vi "Measure vs B2Dv12.vi"() -> ()   [LabVIEW 2009]
doc: "This VI is an example operator panel.\n\nThe VI contains a table for the field values that may be configured manually, or loaded by checking the \"Prompt for File\" box. The data file should contain 3 columns of data, with each column delimited by a tab character.\n\nBefore the VI is executed, set the desired field units and coordinate system. Once the VI is started, follow the directions in the STATUS indicator to operate. Once a field value is achieved, it will be held indefinitely with no user intervention.\n\nThe present field is displayed in the selected units and coordinate system. The present field is queried once per second.\n\nIf a field point is specified that is outside the limits for the magnet, the VI will abort execution."
uses:
  <vilib>/Utility/file.llb/Read From Spreadsheet File (DBL).vi
panel:
  in  "PID off":bool
  in  "Go to zero and SH off":bool=TRUE
  in  "Port Num- TRBridge":string="7"
  in  "GPIB SIM900":string="2"
  in  "TempSensor":bool=TRUE
  in  "AH":bool=TRUE
  in  "GPIB HP 2":string="13"
  in  "Wait between \nVectors":bool
  in  "Change\nPID\n(DetermineSIMPID.vi)":bool
  in  "Wait between \nVectors (ms)":u32=3000
  in  "X Axis":enum16{"B", "phi"}(ring)
  in  "Y Axis":T1(ring)=enum."HP (V)2"
  out "measured data":dbl[][](array[numeric])
  out "XY Graph":T2(graph)
  in  "Notes:":string="Datum: 4.09.12, Uhrzeit: 16:00, Sweep 0.5T/min,(measurevsB2Dv12.vi)), kapazitive Messung, Probe MnSi 30nm auf CuBe Cantilever (SI097) Tset= 40K, tmeasure=ca. 32K, R=1096Ohm ,   Einbauwinkel 15° (optischer Probenstab) ,average time 4," caption="Notizen:"
  out "Messfile Refnum":refnum<file>
  in  "Measurement File":path=path "D:/UserData/Matthias/Messungen/MnSi/120904/SI097_120904_32K_m3.txt"
  in  "Sample name:":string="MnSi 30nm"
  in  "HP 1":bool
  in  "GPIB HP":string="13"
  in  "HP 2":bool
  in  "LI 3":bool
  in  "GPIB L 3":string="8"
  in  "LI 2":bool
  in  "GPIB L 2":string="8"
  in  "LI 1":bool
  in  "GPIB L 1":string="8"
  out "Number of lines":i32=9
  in  "Operation":u16(ring)=1 items=["Stepwise", "Continous"]
  out "Ramp Rate along Vector (T/min)":dbl=0.15000000000000002 format="%.3f"
  out "Current Ramp Rate Z (T/min)":dbl=0.14488663318941059 format="%.3f"
  out "Current Ramp Rate Y (T/min)":dbl=0.03883121840783761 format="%.3f"
  in  "User defined Ramp Rate (T/min)":bool=TRUE
  in  "User defined Ramp Rate (T/min)":dbl=0.15 format="%.3f"
  in  "Z-Axis Communications Config":T3={"GPIB address"=22, "GPIB bus"=1, "connection ID"=refnum, "IP"="111.111.111.1", "Active Comm Interface"=0, "Serial Port"="", "Programmer Type"=0} {"Programmer Type" items=["Model 430", "Model 420"]; "Active Comm Interface" items=["TCP/IP (Model 430 Only)", "RS232", "IEEE488"]}
  in  "Max Ramp Rate - Y Axis (A/s)":dbl=0.055 format="%.3f"
  in  "Max Ramp Rate - Z Axis (A/s)":dbl=0.19 format="%.3f"
  in  "Magnitude Limit (kG)":dbl=45.1 format="%.3f"
  in  "Y-Axis Communications Config":T3={"GPIB address"=22, "GPIB bus"=1, "connection ID"=refnum, "IP"="111.111.111.2", "Active Comm Interface"=0, "Serial Port"="", "Programmer Type"=0} {"Programmer Type" items=["Model 430", "Model 420"]; "Active Comm Interface" items=["TCP/IP (Model 430 Only)", "RS232", "IEEE488"]}
  out "Cartesian Display (T)":T4={"Y-Axis Field (T)"=0.2, "Z-Axis Field (T)"=-1e-05} {"Z-Axis Field (T)" format="%.3f"; "Y-Axis Field (T)" format="%.3f"}
  in  "Starting index":i32=1
  in  "Normal color":u32(colorbox)=11711154
  in  "Highlight color":u32(colorbox)=16711680
  in  "Prompt for File?":bool
  out "Continue Execution?":bool=TRUE
  out "error out":T5
  in  "error in":T5
  out "STATUS":string="Ramping to field vector 1..."
  in  "Ramping Control":u16(ring)=1 items=["NEXT VECTOR", "RAMPING", "HOLDING", "PAUSE", "ZERO"]
  out "Cartesian Display (kG)":T6 {"Z-Axis Field (kG)" format="%.3f"; "Y-Axis Field (kG)" format="%.3f"}
  in  "Field Values":string[][](table)=[["4", "105"], ["0.2", "105"], ["4", "105"], ["0.1", "105"], ["2", "105"], ["-4", "105"], ["-0.2", "105"], ["-4", "105"], ["0", "105"]]
  out "Switch Heaters":bool=TRUE
  out "Polar Display (T)":T7={"q (degrees)"=300.06858282186244, "Field Magnitude (T)"=0.0008781799360040061} {"Field Magnitude (T)" format="%.3f"; "q (degrees)" format="%.3f"}
  out "Polar Display (kG)":T8 {"Field Magnitude (kG)" format="%.3f"; "q (degrees)" format="%.3f"}
  in  "Coordinate System":u16(ring)=1 items=["Cartesian", "Polar"]
  in  "Magnetic Field Units":u16(ring)=1 items=["kG", "Tesla"]
  # "kontinuirliche Messung mit PID off bei 0, geht nur im Cartesian mode!"
  # "Measurement Display"
  # "Measurement Settings"
  # "Magnet Settings"
  # "Max Ramp Rate z: 1.27 T/min\nMax Ramp Rate y: 0.17 T/min"
  # "Devices"
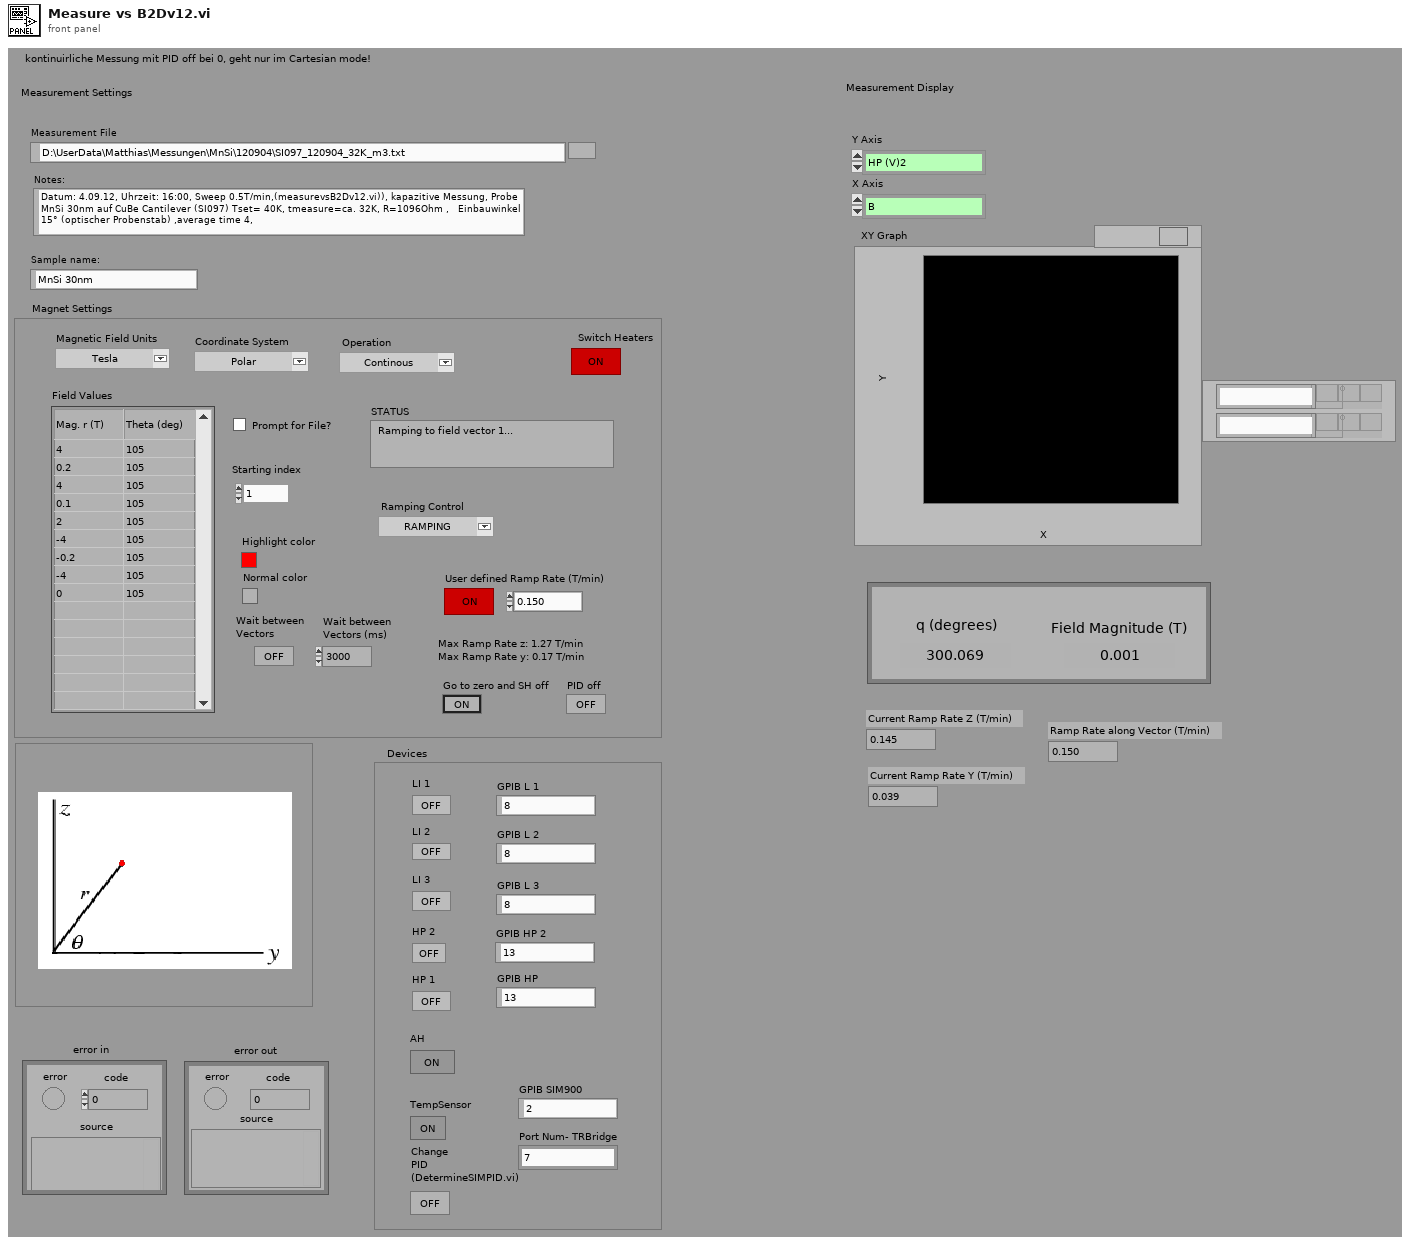
[diagram p1: front panel]
types:
  T1 = enum16{"B", "phi", "LI 1 Vx", "LI 1 Vy", "LI 2 Vx", "LI 2 Vy", "LI 3 Vx", "LI 3 Vy", "LI 4 Vx", "LI 4 Vy", "HP (V)", "HP (V)2", "AH C (pF)", "AH loss", "T (Ohms)", "Timestamp"}
  T2 = cluster{"measured data":dbl[], "measured data":dbl[]}
  T3 = cluster{"GPIB address":i16, "GPIB bus":i16, "connection ID":refnum<k5>, "IP":string, "Active Comm Interface":u16, "Serial Port":refnum<visa-resource-name>, "Programmer Type":u16}
  T4 = cluster{"Y-Axis Field (T)":dbl, "Z-Axis Field (T)":dbl}
  T5 = cluster{"error":bool, "code":i32, "source":string}
  T6 = cluster{"Y-Axis Field (kG)":dbl, "Z-Axis Field (kG)":dbl}
  T7 = cluster{"q (degrees)":dbl, "Field Magnitude (T)":dbl}
  T8 = cluster{"q (degrees)":dbl, "Field Magnitude (kG)":dbl}
  T9 = enum16{"", "RAMPING", "HOLDING", "PAUSED", "MANUAL UP", "MANUAL DOWN", "ZEROING CURRENT", "QUENCH DETECTED", "HEATING SWITCH"}
  T10 = enum16{"", "RAMPING", "HOLDING", "PAUSED", "MANUAL UP", "MANUAL DOWN", "ZEROING CURRENT", "QUENCH DETECTED", "HEATING SWITCH", "AT ZER0", "COOLING SWITCH"}
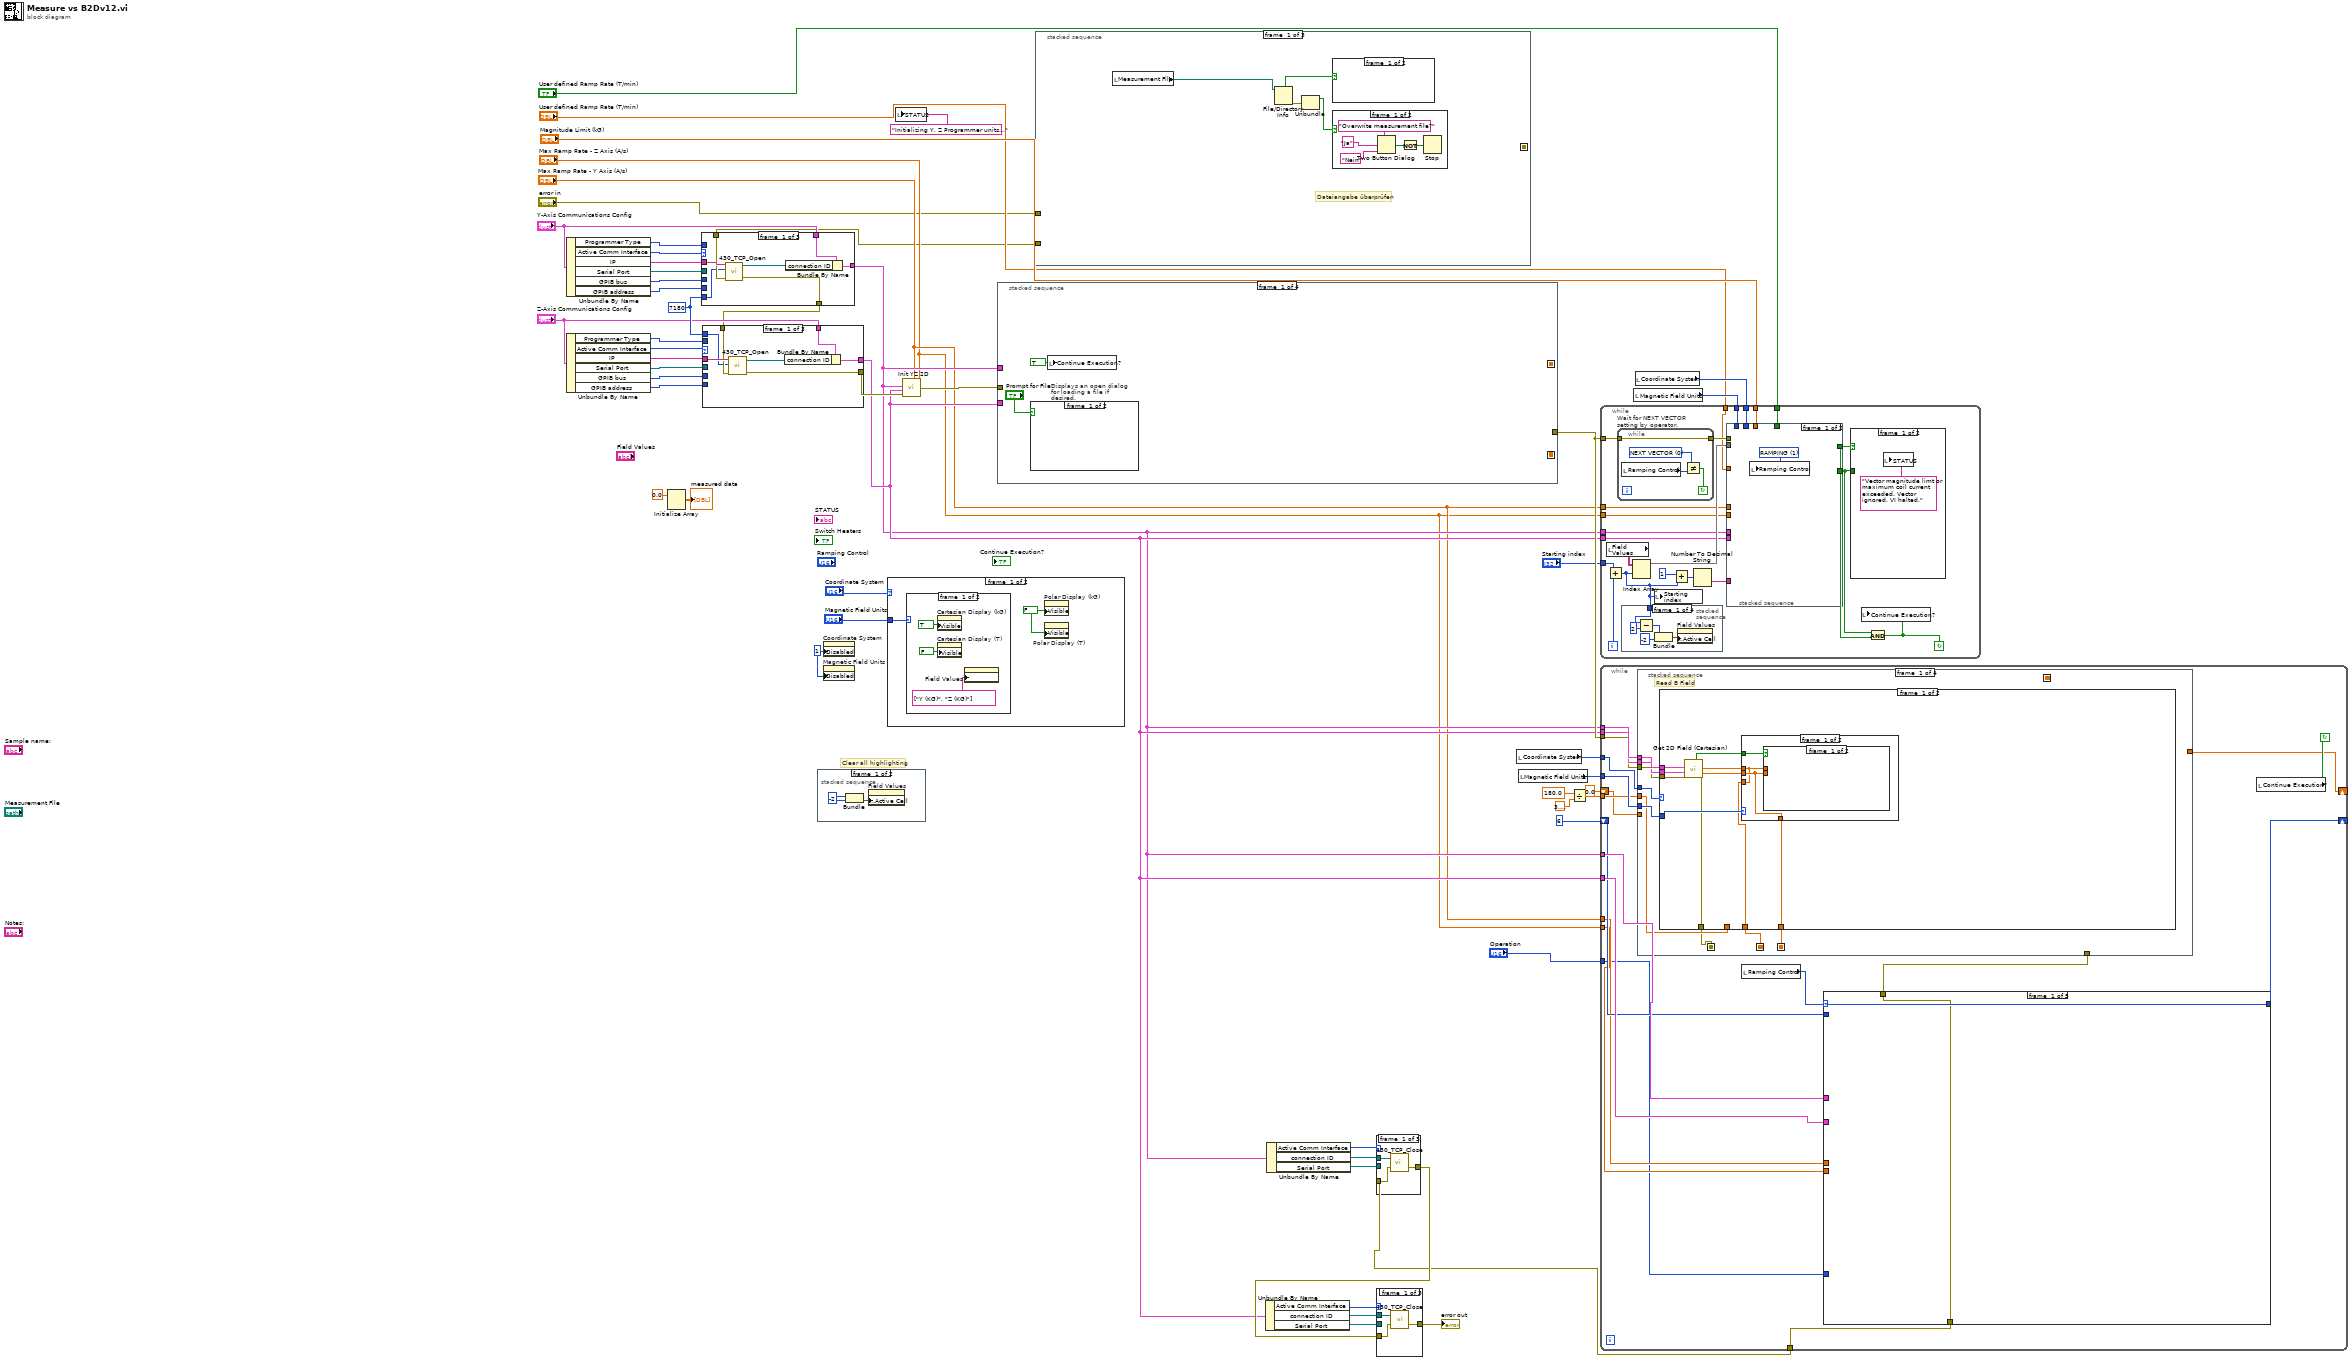
[diagram p0: block diagram]
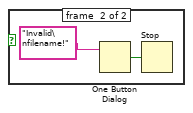
[diagram p3: hidden frame]
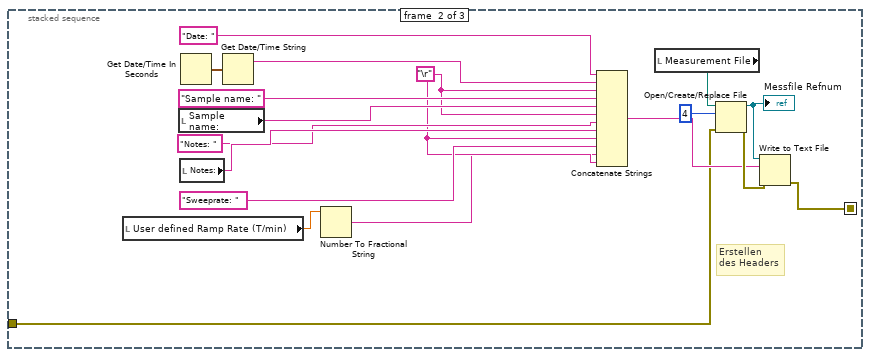
[diagram p4: hidden frame]
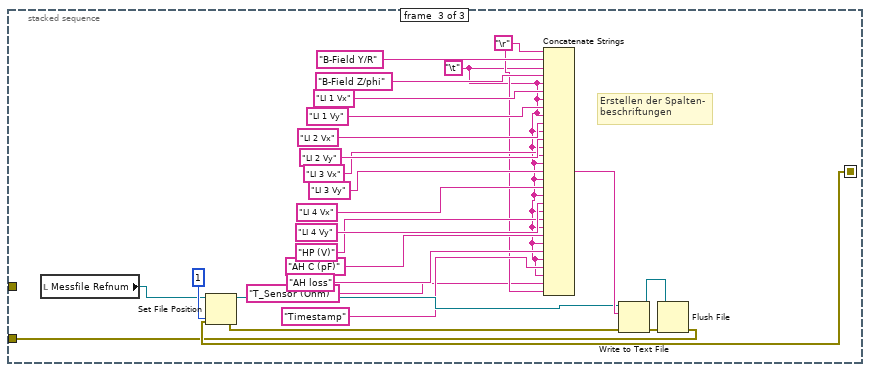
[diagram p5: hidden frame]
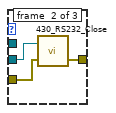
[diagram p6: hidden frame]
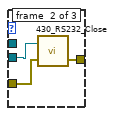
[diagram p8: hidden frame]
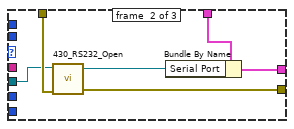
[diagram p10: hidden frame]
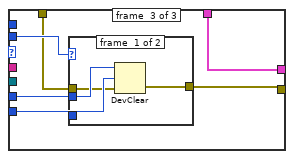
[diagram p11: hidden frame]
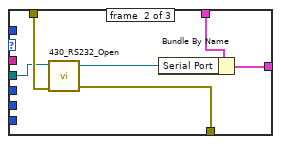
[diagram p13: hidden frame]
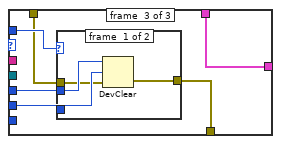
[diagram p14: hidden frame]
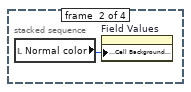
[diagram p16: hidden frame]
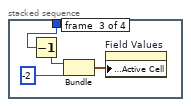
[diagram p17: hidden frame]
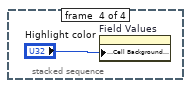
[diagram p18: hidden frame]
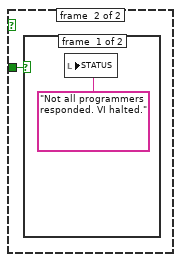
[diagram p19: hidden frame]
diagram:
  w39 = 7180 ("TCP Port")
  w52 = u8 1 ("Write Attribute")
  # "Clear all highlighting"
  n1 = Unbundle By Name("Z-Axis Communications Config") -> ("Programmer Type"=w15:u16, "Active Comm Interface"=w38:u16, "IP"=w35:string, "Serial Port"=w34:refnum<visa-resource-name>, "GPIB bus"=w14:i16, "GPIB address"=w13:i16)
  n2 = Unbundle By Name("Y-Axis Communications Config") -> ("Programmer Type"=w9:u16, "Active Comm Interface"=w37:u16, "IP"=w36:string, "Serial Port"=w33:refnum<visa-resource-name>, "GPIB bus"=w10:i16, "GPIB address"=w11:i16)
  n3 = Initialize Array(0.0 ("element")) -> (→"measured data":dbl[][])  [unwired: 2 in]
  n4 = stacked-sequence {
    frame #0 {
      w55 = -2
      n5 = Bundle(w55, w55) -> (w56:cluster{i32, i32})  [unwired: 1 in]
      n6 = property on="Field Values" class="Tbl (strict)"("Active Cell:Active Cell"=w56) -> ()  [unwired: 2 in, 2 out]
    }
    frame #1 {
      n7 = property on="Field Values" class="Tbl (strict)"("Active Cell:Cell Background Color"="Normal color") -> ()  [unwired: 2 in, 2 out]
    }
  }
  n8 = property on="Coordinate System" class="Ring (strict)"("Disabled"=w52) -> ()  [unwired: 2 in, 2 out]
  n9 = property on="Magnetic Field Units" class="Ring (strict)"("Disabled"=w52) -> ()  [unwired: 2 in, 2 out]
  n10 = case shown="1" "Coordinate System" {
    tunnel: "Magnetic Field Units" -> [w59 w67]
    frame #0 {
      w58 = FALSE ("Write Attribute")
      (unwired) FALSE ("Write Attribute")
      (unwired) TRUE ("Write Attribute")
      n11 = case shown="1" w59 {
        frame #0 {
          n12 = property on="Cartesian Display (kG)" class="Cluster (strict)"("Visible"=TRUE ("Write Attribute")) -> ()  [unwired: 2 in, 2 out]
          n13 = property on="Cartesian Display (T)" class="Cluster (strict)"("Visible"=FALSE ("Write Attribute")) -> ()  [unwired: 2 in, 2 out]
          n14 = property on="Field Values" class="Tbl (strict)"("Column Header Strings[]"=string[] ["Y (KG)", "Z (KG)"] ("Write Attribute")) -> ()  [unwired: 2 in, 2 out]
        }
        frame #1 {
          n15 = property on="Cartesian Display (kG)" class="Cluster (strict)"("Visible"=FALSE ("Write Attribute")) -> ()  [unwired: 2 in, 2 out]
          n16 = property on="Cartesian Display (T)" class="Cluster (strict)"("Visible"=TRUE ("Write Attribute")) -> ()  [unwired: 2 in, 2 out]
          n17 = property on="Field Values" class="Tbl (strict)"("Column Header Strings[]"=string[] ["Y (T)", "Z (T)"] ("Write Attribute")) -> ()  [unwired: 2 in, 2 out]
        }
      }
      n18 = property on="Polar Display (kG)" class="Clust (strict)"("Visible"=w58) -> ()  [unwired: 2 in, 2 out]
      n19 = property on="Polar Display (T)" class="Clust (strict)"("Visible"=w58) -> ()  [unwired: 2 in, 2 out]
    }
    frame #1 {
      (unwired) FALSE ("Write Attribute")
      (unwired) TRUE ("Write Attribute")
      w66 = FALSE ("Write Attribute")
      n20 = case shown="1" w67 {
        frame #0 {
          n21 = property on="Polar Display (kG)" class="Clust (strict)"("Visible"=TRUE ("Write Attribute")) -> ()  [unwired: 2 in, 2 out]
          n22 = property on="Polar Display (T)" class="Clust (strict)"("Visible"=FALSE ("Write Attribute")) -> ()  [unwired: 2 in, 2 out]
          n23 = property on="Field Values" class="Tbl (strict)"("Column Header Strings[]"=string[] ["Mag. r (KG)", "Theta (deg)"] ("Write Attribute")) -> ()  [unwired: 2 in, 2 out]
        }
        frame #1 {
          n24 = property on="Polar Display (kG)" class="Clust (strict)"("Visible"=FALSE ("Write Attribute")) -> ()  [unwired: 2 in, 2 out]
          n25 = property on="Polar Display (T)" class="Clust (strict)"("Visible"=TRUE ("Write Attribute")) -> ()  [unwired: 2 in, 2 out]
          n26 = property on="Field Values" class="Tbl (strict)"("Column Header Strings[]"=string[] ["Mag. r (T)", "Theta (deg)"] ("Write Attribute")) -> ()  [unwired: 2 in, 2 out]
        }
      }
      n27 = property on="Cartesian Display (kG)" class="Cluster (strict)"("Visible"=w66) -> ()  [unwired: 2 in, 2 out]
      n28 = property on="Cartesian Display (T)" class="Cluster (strict)"("Visible"=w66) -> ()  [unwired: 2 in, 2 out]
    }
  }
  n29 = local write "STATUS"("Initializing Y, Z Programmer units..." ("STATUS")) -> ()
  n30 = stacked-sequence {
    seq-local: [_ w85 _] -> [_ _ w110]
    tunnel: "error in" -> [_ w86 _]
    tunnel: [_ _ w109] -> w4
    frame #0 {
      # "Dateiangabe überprüfen"
      n31 = local read "Measurement File"() -> (w77:path)
      n32 = File/Directory Info(path=w77) -> (directory=w75:bool, error out=w76:errorcluster)  [unwired: 1 in, 5 out]
      n33 = Unbundle(w76) -> ("status"=w74:bool)  [unwired: 2 out]
      n34 = case shown="False" w75 {
        frame #0 {
        }
        frame #1 {
          n35 = One Button Dialog(message="Invalid\nfilename!") -> (true=w83:bool)  [unwired: 1 in]
          n36 = Stop(stop? (T)=w83) -> ()
        }
      }
      n37 = case shown="False" w74 {
        frame #0 {
          n38 = Two Button Dialog(message="Overwrite measurement file?", 1:"Nein", 2:"Ja") -> (T button?=w79:bool)
          n39 = Not(x=w79) -> (.not. x?=w78:bool)
          n40 = Stop(stop? (T)=w78) -> ()
        }
        frame #1 {
        }
      }
    }
    frame #1 {
      w89 = "\r"
      # "Erstellen\ndes Headers"
      n41 = local read "User defined Ramp Rate (T/min)"() -> (w88:dbl)
      n42 = local read "Sample name:"() -> (w95:string)
      n43 = local read "Notes:"() -> (w97:string)
      n44 = Get Date/Time In Seconds() -> (seconds since 1Jan1904=w91:timestamp)
      n45 = Get Date/Time String(seconds (now)=w91) -> (date string=w93:string)  [unwired: 2 in, 1 out]
      n46 = Number To Fractional String(number=w88) -> (F-format string=w87:string)  [unwired: 3 in]
      n47 = Concatenate Strings("Date: ", w93, w89, "Sample name: ", w95, w89, "Notes: ", w97, w89, "Sweeprate: ", w87, w89) -> (w101:string)
      n48 = local read "Measurement File"() -> (w98:path)
      n49 = Open/Create/Replace File(file path (use dialog)=w98, error in=w86, operation (0:open)=4) -> (refnum out=w100:refnum<file>, error out=w102:errorcluster)  [unwired: 3 in, 1 out]
      "Messfile Refnum" <- w100
      n50 = Write to Text File(file (use dialog)=w100, text=w101, error in=w102) -> (error out=w85:errorcluster)  [unwired: 1 in, 2 out]
    }
    frame #2 {
      w104 = "\t"
      w105 = "\r"
      # "Erstellen der Spalten-\nbeschriftungen"
      n51 = local read "Messfile Refnum"() -> (w117:refnum<file>)
      n52 = Set File Position(refnum=w117, from (0:start)=1, error in=w110) -> (refnum out=w123:refnum<file>, error out=w125:errorcluster)  [unwired: 1 in]
      n53 = Concatenate Strings(w105, "B-Field Y/R", w104, "B-Field Z/phi", w104, "LI 1 Vx", w104, "LI 1 Vy", w104, "LI 2 Vx", w104, "LI 2 Vy", w104, "LI 3 Vx", w104, "LI 3 Vy", w104, "LI 4 Vx", w104, "LI 4 Vy", w104, "HP (V)", w104, "AH C (pF)" ("string"), w104, "AH loss" ("string"), w104, "Timestamp", w104, "T_Sensor (Ohm)" ("string"), w105) -> (w124:string)
      n54 = Write to Text File(file (use dialog)=w123, text=w124, error in=w125) -> (refnum out=w127:refnum<file>, error out=w126:errorcluster)  [unwired: 1 in, 1 out]
      n55 = Flush File(refnum=w127, error in=w126) -> (error out=w109:errorcluster)  [unwired: 1 out]
    }
  }
  n56 = case shown="0, Default" w37 {
    tunnel: w36 -> [w135 _ _]
    tunnel: w4 -> [w134 w141 w143]
    tunnel: "Y-Axis Communications Config" -> [w133 w136 w147]
    tunnel: [w131 w139 w147] -> w22
    tunnel: [w130 w140 w142] -> w12
    tunnel: w39 -> [w129 _ _]
    tunnel: w33 -> [_ w137 _]
    tunnel: w11 -> [_ _ w146]
    tunnel: w10 -> [_ _ w145]
    tunnel: w9 -> [_ _ w144]
    frame #0 {
      n57 = call <userlib>:"430_TCP_Open.vi"("IP Address"=w135, "TCP Port"=w129, "error in (no error)"=w134) -> ("connection ID"=w132:refnum<k5>, "error out"=w130:errorcluster)  [unwired: 3 in, 1 out]
      n58 = Bundle By Name(cluster=w133, "connection ID"=w132) -> (w131:T3)
    }
    frame #1 {
      n59 = call <userlib>:"430_RS232_Open.vi"("VISA resource name"=w137, "error in (no error)"=w141) -> ("VISA resource name out"=w138:refnum<visa-resource-name>, "error out"=w140:errorcluster)  [unwired: 5 in]
      n60 = Bundle By Name(cluster=w136, "Serial Port"=w138) -> (w139:T3)
    }
    frame #2 {
      n61 = case shown="1" w144 {
        tunnel: w145 -> [w151 _]
        tunnel: w146 -> [w150 _]
        tunnel: w143 -> [w149 w152]
        tunnel: [w148 w152] -> w142
        frame #0 {
          n62 = DevClear(2:w149, 3:w150, 4:w151) -> (0:w148:errorcluster)  [unwired: 1 out]
        }
        frame #1 {
        }
      }
    }
  }
  n63 = case shown="0, Default" w38 {
    tunnel: w35 -> [w159 _ _]
    tunnel: w12 -> [w158 w165 w167]
    tunnel: [w157 w164 w166] -> w32
    tunnel: "Z-Axis Communications Config" -> [w156 w162 w171]
    tunnel: [w154 w163 w171] -> w23
    tunnel: w39 -> [w153 _ _]
    tunnel: w34 -> [_ w160 _]
    tunnel: w15 -> [_ _ w170]
    tunnel: w14 -> [_ _ w169]
    tunnel: w13 -> [_ _ w168]
    frame #0 {
      n64 = call <userlib>:"430_TCP_Open.vi"("IP Address"=w159, "TCP Port"=w153, "error in (no error)"=w158) -> ("connection ID"=w155:refnum<k5>, "error out"=w157:errorcluster)  [unwired: 3 in, 1 out]
      n65 = Bundle By Name(cluster=w156, "connection ID"=w155) -> (w154:T3)
    }
    frame #1 {
      n66 = call <userlib>:"430_RS232_Open.vi"("VISA resource name"=w160, "error in (no error)"=w165) -> ("VISA resource name out"=w161:refnum<visa-resource-name>, "error out"=w164:errorcluster)  [unwired: 5 in]
      n67 = Bundle By Name(cluster=w162, "Serial Port"=w161) -> (w163:T3)
    }
    frame #2 {
      n68 = case shown="0, Default" w170 {
        tunnel: w169 -> [w175 _]
        tunnel: w168 -> [w174 _]
        tunnel: w167 -> [w173 w176]
        tunnel: [w172 w176] -> w166
        frame #0 {
          n69 = DevClear(2:w173, 3:w174, 4:w175) -> (0:w172:errorcluster)  [unwired: 1 out]
        }
        frame #1 {
        }
      }
    }
  }
  n70 = call <userlib>:"Init YZ 2D.vi"("Max Ramp Rate Z-axis"="Max Ramp Rate - Z Axis (A/s)", "Max Ramp Rate Y-axis"="Max Ramp Rate - Y Axis (A/s)", "error in"=w32, "Z-Axis Communications Config"=w23, "Y-Axis Communications Config"=w22) -> ("error out"=w50:T5)  [unwired: 5 in]
  n71 = stacked-sequence {
    seq-local: [_ w184 _ _] -> [_ _ w231 _]
    seq-local: [_ w183 _ _] -> [_ _ w230 _]
    tunnel: w23 -> [_ w186 _ _]
    tunnel: w50 -> [_ w187 _ _]
    tunnel: [_ w182 _ _] -> w46
    tunnel: w22 -> [_ w185 _ _]
    frame #0 {
      n72 = case "Displays an open dialog for loading a file if desired." shown="True" "Prompt for File?" {
        frame #0 {
        }
        frame #1 {
          n73 = call-poly <vilib>:"Read From Spreadsheet File.vi"() -> ("all rows"=w181:dbl[][])  [unwired: 7 in, 4 out]
          n74 = Number To Fractional String(number=w181, precision (6)=i16 4) -> (F-format string=w180:string[][])  [unwired: 2 in]
          n75 = local write "Field Values"(w180) -> ()
        }
      }
      n76 = local write "Continue Execution?"(TRUE ("Continue Execution?")) -> ()
    }
    frame #1 {
      w195 = u16 3 items=["NEXT VECTOR", "RAMPING", "HOLDING", "PAUSE", "ZERO"] ("Ramping Control")
      n77 = call <userlib>:"Get Switch Present.vi"("error in"=w187, "Communications Config"=w185) -> ("error out"=w191:T5, "Switch Present?"=w192:bool)
      n78 = case shown="True" w192 {
        tunnel: w191 -> [w213 w222]
        tunnel: w185 -> [_ w215]
        tunnel: [0.0 w219] -> w183
        tunnel: [w213 w221] -> w190
        frame #0 {
        }
        frame #1 {
          n79 = call <userlib>:"Get Switch Heater Time.vi"("error in"=w222, "Communications Config"=w215) -> ("error out"=w218:T5, "Switch Heating Time (secs)"=w220:dbl)
          n80 = call <userlib>:"Get Switch Heater.vi"("error in"=w218, "Communications Config"=w215) -> ("error out"=w217:T5, "Switch Heater Indicator"=w216:bool)
          n81 = case shown="False" w216 {
            tunnel: [w227 w228] -> w221
            tunnel: w220 -> [w225 _]
            tunnel: [w225 0.0] -> w219
            tunnel: w217 -> [w223 w228]
            tunnel: w215 -> [w224 _]
            frame #0 {
              n82 = call <userlib>:"Set Switch Heater.vi"("error in"=w223, "Switch Heater Control"=TRUE, "Communications Config"=w224) -> ("error out"=w227:T5)
            }
            frame #1 {
            }
          }
        }
      }
      n83 = call <userlib>:"Get Switch Present.vi"("error in"=w190, "Communications Config"=w186) -> ("error out"=w188:T5, "Switch Present?"=w189:bool)
      n84 = case shown="True" w189 {
        tunnel: w188 -> [w196 w205]
        tunnel: w186 -> [_ w198]
        tunnel: [0.0 w202] -> w184
        tunnel: [w196 w204] -> w182
        frame #0 {
        }
        frame #1 {
          n85 = call <userlib>:"Get Switch Heater Time.vi"("error in"=w205, "Communications Config"=w198) -> ("error out"=w201:T5, "Switch Heating Time (secs)"=w203:dbl)
          n86 = call <userlib>:"Get Switch Heater.vi"("error in"=w201, "Communications Config"=w198) -> ("error out"=w200:T5, "Switch Heater Indicator"=w199:bool)
          n87 = case shown="False" w199 {
            tunnel: [w206 w211] -> w204
            tunnel: w203 -> [w209 _]
            tunnel: [w209 0.0] -> w202
            tunnel: w200 -> [w207 w211]
            tunnel: w198 -> [w208 _]
            frame #0 {
              n88 = call <userlib>:"Set Switch Heater.vi"("error in"=w207, "Switch Heater Control"=TRUE, "Communications Config"=w208) -> ("error out"=w206:T5)
            }
            frame #1 {
            }
          }
        }
      }
      n89 = local write "Ramping Control"(w195) -> ()
      n90 = local write "Switch Heaters"(TRUE ("Switch Heater Control")) -> ()
      n91 = property on="Switch Heaters" class="Boolean (strict)"("Disabled"=u8 1 ("Write Attribute")) -> ()  [unwired: 2 in, 2 out]
    }
    frame #2 {
      n92 = Max & Min(x=w231, y=w230) -> (max(x,y)=w232:dbl)  [unwired: 1 out]
      n93 = local write "STATUS"("Heating switches..." ("STATUS")) -> ()
      n94 = Add(x=w232, y=2) -> (x+y=w236:dbl)
      n95 = property on="Ramping Control" class="Ring (strict)"("Disabled"=u8 1 ("Write Attribute")) -> ()  [unwired: 2 in, 2 out]
      n96 = Multiply(x=w236, y=1000) -> (x*y=w235:dbl)
      n97 = Wait (ms)(milliseconds to wait=w235) -> ()  [unwired: 1 out]
    }
    frame #3 {
      n98 = property on="Ramping Control" class="Ring (strict)"("Disabled"=u8 0 ("Write Attribute")) -> ()  [unwired: 2 in, 2 out]
      n99 = local write "STATUS"("Ready to ramp to first vector. Set Ramping Mode to NEXT VECTOR to begin." ("STATUS")) -> ()
      n100 = local read "Field Values"() -> (w241:string[][])
      n101 = Array Size(array=w241) -> (size(s)=w240:i32[])
      n102 = Index Array(array=w240, index=0) -> (element=→"Number of lines":i32)
    }
  }
  n103 = Unbundle By Name(w23) -> ("Active Comm Interface"=w29:u16, "connection ID"=w28:refnum<k5>, "Serial Port"=w27:refnum<visa-resource-name>)
  n104 = Unbundle By Name(w22) -> ("Active Comm Interface"=w30:u16, "connection ID"=w26:refnum<k5>, "Serial Port"=w25:refnum<visa-resource-name>)
  n105 = local read "Coordinate System"() -> (w47:u16)
  n106 = local read "Magnetic Field Units"() -> (w45:u16)
  n107 = Divide(x=180.0, y=3.141592653589793) -> (x/y=w42:dbl)
  n108 = while {
    shift-left: u16 6 ("Ramping Control") -> [w251]
    shift-right: [w252] -> _
    tunnel: [w254] -> w24
    tunnel: w23 -> [w255]
    tunnel: w22 -> [w256]
    tunnel: w42 -> [w258]
    tunnel: w45 -> [w259]
    tunnel: w46 -> [w260]
    tunnel: w23 -> [w261]
    tunnel: w22 -> [w262]
    tunnel: w47 -> [w263]
    tunnel: "Max Ramp Rate - Y Axis (A/s)" -> [w250]
    tunnel: "Max Ramp Rate - Z Axis (A/s)" -> [w249]
    tunnel: "Operation" -> [w248]
    shift-right: [w246] -> _
    shift-left: 0.0 -> [w245]
    stop <- w253 continue-if-true
    n109 = stacked-sequence {
      seq-local: [w266 _ _ _] -> [_ _ w391 _]
      seq-local: [w265 _ _ _] -> [_ w339 w388 _]
      seq-local: [w264 _ _ _] -> [_ w340 w389 _]
      seq-local: [_ _ w376 _] -> [_ _ _ w468]
      tunnel: w263 -> [w272 _ _ w466]
      tunnel: w262 -> [w271 _ _ _]
      tunnel: w261 -> [w270 _ _ _]
      tunnel: w260 -> [w269 _ _ _]
      tunnel: w259 -> [w268 _ _ _]
      tunnel: w258 -> [w267 _ _ _]
      tunnel: [_ _ w390 _] -> w247
      tunnel: [_ w342 _ _] -> w246
      tunnel: w245 -> [_ w341 _ _]
      frame #0 {
        # "Read B Field"
        n110 = case shown="0, Default" w272 {
          tunnel: w271 -> [w282 w305]
          tunnel: w270 -> [w281 w304]
          tunnel: w269 -> [w280 w303]
          tunnel: w268 -> [w279 w302]
          tunnel: w267 -> [_ w301]
          tunnel: [w275 w300] -> w266
          tunnel: [w274 w298] -> w265
          tunnel: [w273 w299] -> w264
          frame #0 {
            n111 = call <userlib>:"Get 2D Field (Cartesian).vi"("Y-Axis Communications Config"=w282, "Z-Axis Communications Config"=w281, "error in"=w280) -> ("All Instruments Responded?"=w276:bool, "Y-Axis Field (kG)"=w278:dbl, "Z-Axis Field (kG)"=w277:dbl, "error out"=w275:T5)  [unwired: 2 in]
            n112 = case shown="0, Default" w279 {
              tunnel: w278 -> [w283 w291]
              tunnel: w277 -> [w284 w292]
              tunnel: w276 -> [w285 w294]
              tunnel: [w284 w290] -> w274
              tunnel: [w283 w289] -> w273
              frame #0 {
                n113 = case shown="True" w285 {
                  tunnel: w283 -> [_ w287]
                  tunnel: w284 -> [_ w286]
                  frame #0 {
                  }
                  frame #1 {
                    n114 = Bundle("Y-Axis Field (kG)"=w287, "Z-Axis Field (kG)"=w286) -> (→"Cartesian Display (kG)":T6)  [unwired: 1 in]
                  }
                }
              }
              frame #1 {
                w293 = 0.1 ("y")
                n115 = Multiply(x=w291, y=w293) -> (x*y=w289:dbl)
                n116 = Multiply(x=w292, y=w293) -> (x*y=w290:dbl)
                n117 = case shown="True" w294 {
                  tunnel: w289 -> [_ w297]
                  tunnel: w290 -> [_ w296]
                  frame #0 {
                  }
                  frame #1 {
                    n118 = Bundle(w297, w296) -> (→"Cartesian Display (T)":cluster{dbl, dbl})  [unwired: 1 in]
                  }
                }
              }
            }
          }
          frame #1 {
            n119 = stacked-sequence {
              tunnel: w305 -> [w316]
              tunnel: w304 -> [w315]
              tunnel: w303 -> [w314]
              tunnel: w302 -> [w313]
              tunnel: w301 -> [w310]
              tunnel: [w308] -> w300
              tunnel: [w307] -> w298
              tunnel: [w306] -> w299
              frame #0 {
                # "Field"
                n120 = call <userlib>:"Get 2D Field (Polar).vi"("Y-Axis Communications Config"=w316, "Z-Axis Communications Config"=w315, "error in"=w314) -> ("All Instruments Responded?"=w309:bool, "Radial (r) Field (kG)"=w312:dbl, "q (radians)"=w311:dbl, "error out"=w308:T5)  [unwired: 2 in]
                n121 = case shown="1" w313 {
                  tunnel: w312 -> [w318 w330]
                  tunnel: w311 -> [w320 w329]
                  tunnel: w310 -> [w319 w328]
                  tunnel: w309 -> [w321 w327]
                  tunnel: [w318 w325] -> w307
                  tunnel: [w317 w326] -> w306
                  frame #0 {
                    n122 = Multiply(x=w320, y=w319) -> (x*y=w317:dbl)
                    n123 = case shown="True" w321 {
                      tunnel: w318 -> [_ w322]
                      tunnel: w317 -> [_ w323]
                      frame #0 {
                      }
                      frame #1 {
                        n124 = Bundle(w323, "Radial (r) Field (kG)"=w322) -> (→"Polar Display (kG)":cluster{dbl, "Radial (r) Field (kG)":dbl})  [unwired: 1 in]
                      }
                    }
                  }
                  frame #1 {
                    n125 = Multiply(x=w330, y=0.1) -> (x*y=w326:dbl)
                    n126 = Multiply(x=w329, y=w328) -> (x*y=w325:dbl)
                    n127 = case shown="True" w327 {
                      tunnel: w326 -> [_ w332]
                      tunnel: w325 -> [_ w333]
                      frame #0 {
                      }
                      frame #1 {
                        n128 = Bundle(w333, w332) -> (→"Polar Display (T)":cluster{dbl, dbl})  [unwired: 1 in]
                      }
                    }
                  }
                }
              }
            }
          }
        }
      }
      frame #1 {
        # "Change PID"
        n129 = Square(x=w340) -> (x^2=w337:dbl)
        n130 = Square(x=w339) -> (x^2=w338:dbl)
        n131 = Add(x=w337, y=w338) -> (x+y=w336:dbl)
        n132 = Square Root(x=w336) -> (sqrt(x)=w335:dbl)
        n133 = case shown="True" "Change\nPID\n(DetermineSIMPID.vi)" {
          tunnel: w335 -> [_ w354]
          tunnel: [_ w350] -> w342
          tunnel: w341 -> [_ w352]
          frame #0 {
          }
          frame #1 {
            n134 = Absolute Value(x=w354) -> (abs(x)=w350:dbl)
            n135 = Less Or Equal?(x=w350, y=0.07 ("upper limit")) -> (x <= y?=w347:bool)
            n136 = Greater?(x=w352, y=0.07 ("upper limit")) -> (0:w348:bool)
            n137 = Not(x=w348) -> (.not. x?=w345:bool)
            n138 = Not(x=w347) -> (.not. x?=w346:bool)
            n139 = And(x=w348, y=w347) -> (x .and. y?=w353:bool)
            n140 = And(x=w345, y=w346) -> (x .and. y?=w344:bool)
            n141 = case shown="True" w353 {
              frame #0 {
              }
              frame #1 {
                n142 = stacked-sequence {
                  frame #0 {
                    n143 = call "SIM960Poff.vi"("off/on (0/1)"="0", "Port Num- PID"="1", "GPIB-Adress"="2") -> ()  [unwired: 9 in]
                  }
                  frame #1 {
                    n144 = call "SIM960Poff.vi"("off/on (0/1)"="0", "Port Num- PID"="3", "GPIB-Adress"="2") -> ()  [unwired: 9 in]
                  }
                  frame #2 {
                    n145 = call "SIM960ChangeSignP.vi"("Port Num- PID"="1", "GPIB-Adress"="2") -> ()  [unwired: 10 in]
                  }
                }
              }
            }
            n146 = case shown="True" w344 {
              frame #0 {
              }
              frame #1 {
                n147 = stacked-sequence {
                  frame #0 {
                    n148 = call "SIM960Poff.vi"("off/on (0/1)"="1", "Port Num- PID"="3", "GPIB-Adress"="2") -> ()  [unwired: 9 in]
                  }
                  frame #1 {
                    n149 = call "SIM960Poff.vi"("off/on (0/1)"="1", "Port Num- PID"="1", "GPIB-Adress"="2") -> ()  [unwired: 9 in]
                  }
                }
              }
            }
          }
        }
      }
      frame #2 {
        w375 = u16 2 items=["NEXT VECTOR", "RAMPING", "HOLDING", "PAUSE", "ZERO"] ("Ramping Control")
        # "Zeile in Datei schreiben"
        # "Read and Save Devices"
        n150 = stacked-sequence {
          tunnel: [w403 _ _ _ _ _ _ _] -> w387
          tunnel: [w402 _ _ _ _ _ _ _] -> w386
          tunnel: [_ w416 _ _ _ _ _ _] -> w383
          tunnel: [_ w414 _ _ _ _ _ _] -> w382
          tunnel: [_ _ w426 _ _ _ _ _] -> w381
          tunnel: [_ _ w425 _ _ _ _ _] -> w380
          tunnel: [_ _ _ w437 _ _ _ _] -> w379
          tunnel: [_ _ _ 0.0 _ _ _ _] -> w378
          tunnel: [_ _ _ _ w443 _ _ _] -> w377
          tunnel: [_ _ _ _ _ _ _ w462] -> w370
          tunnel: [_ _ _ _ _ w450 _ _] -> w372
          tunnel: [_ _ _ _ _ w449 _ _] -> w371
          tunnel: [_ _ _ _ _ _ w455 _] -> w369
          frame #0 {
            n151 = case shown="True" "LI 1" {
              tunnel: ["0" ("Antwort2") w410] -> w405
              tunnel: ["0" ("Antwort1") w409] -> w404
              frame #0 {
              }
              frame #1 {
                n152 = call "LI-Ansteuerung.vi"("Frage2"="OUTP? 2", "Frage1"="OUTP? 1", "address string"="GPIB L 1") -> ("Antwort2"=w410:string, "Antwort1"=w409:string)
              }
            }
            n153 = Fract/Exp String To Number(string=w405) -> (number=w402:dbl)  [unwired: 3 in, 1 out]
            n154 = Fract/Exp String To Number(string=w404) -> (number=w403:dbl)  [unwired: 3 in, 1 out]
          }
          frame #1 {
            n155 = case shown="True" "LI 2" {
              tunnel: [w419 w421] -> w415
              tunnel: [w419 w420] -> w417
              frame #0 {
                w419 = "0" ("Antwort1")
              }
              frame #1 {
                n156 = call "LI-Ansteuerung.vi"("Frage2"="OUTP? 2", "Frage1"="OUTP? 1", "address string"="GPIB L 2") -> ("Antwort2"=w421:string, "Antwort1"=w420:string)
              }
            }
            n157 = Fract/Exp String To Number(string=w415) -> (number=w414:dbl)  [unwired: 3 in, 1 out]
            n158 = Fract/Exp String To Number(string=w417) -> (number=w416:dbl)  [unwired: 3 in, 1 out]
          }
          frame #2 {
            n159 = case shown="True" "LI 3" {
              tunnel: [w430 w432] -> w427
              tunnel: [w430 w431] -> w428
              frame #0 {
                w430 = "0" ("Antwort1")
              }
              frame #1 {
                n160 = call "LI-Ansteuerung.vi"("Frage2"="OUTP? 2", "Frage1"="OUTP? 1", "address string"="GPIB L 3") -> ("Antwort2"=w432:string, "Antwort1"=w431:string)
              }
            }
            n161 = Fract/Exp String To Number(string=w428) -> (number=w426:dbl)  [unwired: 3 in, 1 out]
            n162 = Fract/Exp String To Number(string=w427) -> (number=w425:dbl)  [unwired: 3 in, 1 out]
          }
          frame #3 {
            n163 = case shown="True" "HP 2" {
              tunnel: [0.0 ("Voltage") w440] -> w437
              frame #0 {
              }
              frame #1 {
                n164 = call "HP-ReadVoltagev2.vi"("String"="meas:volt:dc? 10,0.001", "HP-Mulitmeter\nGPIB Address"="GPIB HP 2") -> ("Voltage"=w440:dbl)  [unwired: 9 in]
              }
            }
          }
          frame #4 {
            n165 = case shown="False" "HP 1" {
              tunnel: [0.0 ("Voltage") w447] -> w443
              frame #0 {
              }
              frame #1 {
                n166 = call "HP-ReadVoltagev2.vi"("String"="meas:volt:dc? 200,0.001", "HP-Mulitmeter\nGPIB Address"="GPIB HP") -> ("Voltage"=w447:dbl)  [unwired: 9 in]
              }
            }
          }
          frame #5 {
            n167 = case shown="True" "AH" {
              tunnel: [w452 w454] -> w449
              tunnel: [w452 w453] -> w450
              frame #0 {
                w452 = 0.0 ("Voltage")
              }
              frame #1 {
                n168 = call "AHRead2550.vi"() -> ("loss"=w454:dbl, "capacitance"=w453:dbl)  [unwired: 9 in, 1 out]
              }
            }
          }
          frame #6 {
            n169 = case shown="False" "TempSensor" {
              tunnel: [0.0 ("Voltage") w458] -> w455
              frame #0 {
              }
              frame #1 {
                n170 = call "Read_R_Bridge_new_v3.vi"("Port Num- TRBridge"="Port Num- TRBridge", "GPIB-Adress"="GPIB SIM900") -> ("R out"=w459:string)  [unwired: 8 in, 1 out]
                n171 = Fract/Exp String To Number(string=w459) -> (number=w458:dbl)  [unwired: 3 in, 1 out]
              }
            }
          }
          frame #7 {
            n172 = Get Date/Time In Seconds() -> (seconds since 1Jan1904=w463:timestamp)
            n173 = To Double Precision Float(number=w463) -> (double precision float=w462:dbl)
          }
        }
        n174 = local read "Ramping Control"() -> (w374:u16)
        n175 = Build Array(w389, w388, w387, w386, w383, w382, w380, w381, w379, w378, w377, w372, w371, w369, w370) -> (w376:dbl[])
        n176 = Array To Spreadsheet String(array=w376, 3:"%.8f" ("format string")) -> (spreadsheet string=w385:string)  [unwired: 1 in]
        n177 = Equal?(x=w374, y=w375) -> (x = y?=w373:bool)
        n178 = case shown="False" w373 {
          tunnel: w391 -> [w400 w401]
          tunnel: [w399 w401] -> w390
          tunnel: w385 -> [w398 _]
          frame #0 {
            n179 = local read "Messfile Refnum"() -> (w392:refnum<file>)
            n180 = Set File Position(refnum=w392, from (0:start)=1, error in=w400) -> (refnum out=w394:refnum<file>, error out=w395:errorcluster)  [unwired: 1 in]
            n181 = Write to Text File(file (use dialog)=w394, text=w398, error in=w395) -> (refnum out=w397:refnum<file>, error out=w396:errorcluster)  [unwired: 1 in, 1 out]
            n182 = Flush File(refnum=w397, error in=w396) -> (error out=w399:errorcluster)  [unwired: 1 out]
          }
          frame #1 {
          }
        }
      }
      frame #3 {
        n183 = local read "measured data"() -> (w469:dbl[][])
        n184 = Insert Into Array(array=w469, new element=w468) -> (w467:dbl[][])  [unwired: 2 in]
        n185 = case shown="0, Default" w466 {
          tunnel: w467 -> [w485 w499]
          tunnel: "Y Axis" -> [w487 w498]
          tunnel: "X Axis" -> [w475 w497]
          frame #0 {
            n186 = Index Array(array=w485, index (col)=1 ("disabled index (col)")) -> (element=w480:dbl[])  [unwired: 1 in]
            n187 = Index Array(array=w485, index (col)=0 ("disabled index (col)")) -> (element=w479:dbl[])  [unwired: 1 in]
            n188 = Square(x=w480) -> (x^2=w482:dbl[])
            n189 = Square(x=w479) -> (x^2=w483:dbl[])
            n190 = Index Array(array=w485, index (col)=w487) -> (element=w474:dbl[])  [unwired: 1 in]
            n191 = Divide(x=w480, y=w479) -> (x/y=w471:dbl[])
            n192 = Add(x=w483, y=w482) -> (x+y=w481:dbl[])
            n193 = Inverse Tangent(1:w471) -> (0:w470:dbl[])
            n194 = Square Root(x=w481) -> (sqrt(x)=w472:dbl[])
            n195 = Divide(x=w470, y=3.141592653589793) -> (x/y=w477:dbl[])
            n196 = Multiply(x=w477, y=180) -> (x*y=w473:dbl[])
            n197 = case shown="\"B\", Default" w475 {
              tunnel: w474 -> [w490 w493]
              tunnel: w473 -> [_ w492]
              tunnel: w472 -> [w489 _]
              frame #0 {
                n198 = Bundle(w489, "measured data"=w490) -> (w488:cluster{dbl[], "measured data":dbl[]})  [unwired: 1 in]
                n199 = local write "XY Graph"(w488) -> ()
              }
              frame #1 {
                n200 = Bundle(w492, "measured data"=w493) -> (w491:cluster{dbl[], "measured data":dbl[]})  [unwired: 1 in]
                n201 = local write "XY Graph"(w491) -> ()
              }
            }
          }
          frame #1 {
            n202 = Index Array(array=w499, index (col)=w497) -> (element=w496:dbl[])  [unwired: 1 in]
            n203 = Index Array(array=w499, index (col)=w498) -> (element=w495:dbl[])  [unwired: 1 in]
            n204 = Bundle("measured data"=w496, "measured data"=w495) -> (w494:T2)  [unwired: 1 in]
            n205 = local write "XY Graph"(w494) -> ()
          }
        }
        n206 = local write "measured data"(w467) -> ()
      }
    }
    n207 = local read "Ramping Control"() -> (w257:u16)
    n208 = case shown="4" w257 {
      selector: w257 -> [w501 w521 w606 w610 w625]
      tunnel: w256 -> [_ w506 _ w613 w630]
      tunnel: w255 -> [_ w505 _ w612 w629]
      tunnel: [w500 w503 w605 w611 w628] -> w254
      tunnel: [w501 w521 w606 w610 w625] -> w252
      tunnel: w251 -> [_ _ _ w609 w627]
      tunnel: w250 -> [_ _ _ _ w624]
      tunnel: w249 -> [_ _ _ _ w623]
      tunnel: w248 -> [_ w513 _ _ _]
      tunnel: w247 -> [w500 w509 w605 w607 w622]
      frame #0 {
      }
      frame #1 {
        w516 = T9."HOLDING" ("y")
        n209 = local read "Number of lines"() -> (w510:i32)
        n210 = local read "Starting index"() -> (w512:i32)
        n211 = call <userlib>:"Get Ramping Mode.vi"("Communications Config"=w506, "error in"=w509) -> ("Ramping Mode"=w519:T10, "error out"=w520:T5)  [unwired: 1 out]
        n212 = call <userlib>:"Get Ramping Mode.vi"("Communications Config"=w505, "error in"=w520) -> ("Ramping Mode"=w518:T10, "error out"=w504:T5)  [unwired: 1 out]
        n213 = Less?(x=w512, y=w510) -> (x < y?=w511:bool)
        n214 = Equal?(x=w519, y=w516) -> (x = y?=w515:bool)
        n215 = Equal?(x=w518, y=w516) -> (x = y?=w514:bool)
        n216 = Compound Arithmetic op=AND(w515, w514) -> (w517:bool)
        n217 = case shown="True" w517 {
          tunnel: w513 -> [_ w531]
          tunnel: w511 -> [_ w530]
          tunnel: "Wait between \nVectors (ms)" -> [_ w529]
          tunnel: "Wait between \nVectors" -> [_ w528]
          tunnel: w506 -> [_ w526]
          tunnel: w505 -> [_ w525]
          tunnel: w504 -> [w522 w524]
          tunnel: [w522 w523] -> w503
          tunnel: "Go to zero and SH off" -> [_ w527]
          frame #0 {
          }
          frame #1 {
            n218 = case shown="1" w531 {
              tunnel: w530 -> [_ w542]
              tunnel: w529 -> [_ w541]
              tunnel: w528 -> [_ w540]
              tunnel: w527 -> [_ w539]
              tunnel: w526 -> [_ w538]
              tunnel: w525 -> [_ w537]
              tunnel: w524 -> [w532 w536]
              tunnel: [w532 w535] -> w523
              frame #0 {
                w534 = u16 2 items=["NEXT VECTOR", "RAMPING", "HOLDING", "PAUSE", "ZERO"] ("Ramping Control")
                n219 = local write "STATUS"("Holding at current vector. Set Ramping Mode to NEXT VECTOR to continue." ("STATUS")) -> ()
                n220 = local write "Ramping Control"(w534) -> ()
              }
              frame #1 {
                # "Go to NEXT VECTOR automatically"
                n221 = case shown="False" w542 {
                  tunnel: w541 -> [_ w599]
                  tunnel: w540 -> [_ w598]
                  tunnel: w539 -> [w547 _]
                  tunnel: w538 -> [w546 _]
                  tunnel: w537 -> [w545 _]
                  tunnel: w536 -> [w544 w597]
                  tunnel: [w543 w597] -> w535
                  frame #0 {
                    n222 = case shown="True" w547 {
                      tunnel: [w548 w552] -> w543
                      tunnel: w546 -> [_ w551]
                      tunnel: w545 -> [_ w550]
                      tunnel: w544 -> [w548 w549]
                      frame #0 {
                      }
                      frame #1 {
                        n223 = stacked-sequence {
                          seq-local: [_ _ w569 _ _ _ _] -> [_ _ _ _ w590 _ _]
                          tunnel: [_ _ _ _ w588 _ _] -> w552
                          tunnel: w551 -> [_ w556 w568 _ _ _ _]
                          tunnel: w550 -> [_ w555 w567 _ _ _ _]
                          tunnel: w549 -> [_ _ w566 _ _ _ _]
                          frame #0 {
                            w553 = u16 2 items=["NEXT VECTOR", "RAMPING", "HOLDING", "PAUSE", "ZERO"] ("Ramping Control")
                            n224 = local write "STATUS"("Holding at current vector. Set Ramping Mode to NEXT VECTOR to continue." ("STATUS")) -> ()
                            n225 = local write "Ramping Control"(w553) -> ()
                          }
                          frame #1 {
                            w561 = u16 0 items=["kG", "Tesla"] ("Magnetic Field Units")
                            w560 = u16 0 items=["Cartesian", "Polar"] ("Coordinate System")
                            n226 = Build Array("0", "0") -> (w559:string[])
                            n227 = call <userlib>:"Set 2D Next Vector_entwurf.vi"("Coordinate System"=w560, "Magnetic Field Units"=w561, "Magnitude Limit (kG)"=45.0, "Y-Axis Communications Config"=w556, "Input Vector"=w559, "Z-Axis Communications Config"=w555, "User defined Ramp Rate (T/min)"=FALSE, "Max Ramp Rate - Y Axis (A/s)"=0.05, "Max Ramp Rate - Z Axis (A/s)"=0.15) -> ()  [unwired: 5 in, 6 out]
                          }
                          frame #2 {
                            n228 = while {
                              tunnel: [w573] -> w569
                              tunnel: w568 -> [w572]
                              tunnel: w567 -> [w571]
                              tunnel: w566 -> [w570]
                              stop <- w575 stop-if-true
                              w578 = T9."HOLDING" ("y")
                              n229 = call <userlib>:"Get Ramping Mode.vi"("Communications Config"=w572, "error in"=w570) -> ("Ramping Mode"=w579:T10, "error out"=w581:T5)  [unwired: 1 out]
                              n230 = call <userlib>:"Get Ramping Mode.vi"("Communications Config"=w571, "error in"=w581) -> ("Ramping Mode"=w580:T10, "error out"=w573:T5)  [unwired: 1 out]
                              n231 = Equal?(x=w579, y=w578) -> (x = y?=w577:bool)
                              n232 = Equal?(x=w580, y=w578) -> (x = y?=w576:bool)
                              n233 = Compound Arithmetic op=AND(w577, w576) -> (w575:bool)
                              n234 = Wait (ms)(milliseconds to wait=u32 1000) -> ()  [unwired: 1 out]
                            }
                          }
                          frame #3 {
                            n235 = case shown="True" "PID off" {
                              frame #0 {
                              }
                              frame #1 {
                                w585 = "0" ("off/on (0/1)")
                                w586 = "2" ("GPIB-Adress")
                                n236 = call "SIM960Poff.vi"("off/on (0/1)"=w585, "Port Num- PID"="3", "GPIB-Adress"=w586) -> ()  [unwired: 9 in]
                                n237 = call "SIM960Poff.vi"("off/on (0/1)"=w585, "Port Num- PID"="1", "GPIB-Adress"=w586) -> ()  [unwired: 9 in]
                              }
                            }
                            n238 = Wait (ms)(milliseconds to wait=u32 10000) -> ()  [unwired: 1 out]
                          }
                          frame #4 {
                            w591 = u16 1 items=["RAMP", "PAUSE", "MANUAL UP", "MANUAL DOWN", "ZERO"] ("Ramping Mode")
                            w592 = u16 1 items=["RAMP", "PAUSE", "MANUAL UP", "MANUAL DOWN", "ZERO"] ("Ramping Mode")
                            n239 = call <userlib>:"Set Ramping Mode.vi"("error in"=w590, "Ramping Mode"=w592) -> ("error out"=w589:T5)  [unwired: 1 in]
                            n240 = call <userlib>:"Set Ramping Mode.vi"("error in"=w589, "Ramping Mode"=w591) -> ("error out"=w588:T5)  [unwired: 1 in]
                          }
                          frame #5 {
                            n241 = call <userlib>:"430_TCP_PSoff.vi"("IP Address"="111.111.111.2", "Switch Heater Control"=FALSE) -> ()  [unwired: 5 in, 2 out]
                            n242 = call <userlib>:"430_TCP_PSoff.vi"("IP Address"="111.111.111.1", "Switch Heater Control"=FALSE) -> ()  [unwired: 5 in, 2 out]
                          }
                          frame #6 {
                          }
                        }
                      }
                    }
                  }
                  frame #1 {
                    n243 = stacked-sequence {
                      tunnel: w599 -> [w601 _]
                      tunnel: w598 -> [w600 _]
                      frame #0 {
                        n244 = case shown="True" w600 {
                          tunnel: w601 -> [_ w602]
                          frame #0 {
                          }
                          frame #1 {
                            n245 = Wait (ms)(milliseconds to wait=w602) -> ()  [unwired: 1 out]
                          }
                        }
                      }
                      frame #1 {
                        w604 = u16 0 items=["NEXT VECTOR", "RAMPING", "HOLDING", "PAUSE", "ZERO"] ("Ramping Control")
                        n246 = local write "Ramping Control"(w604) -> ()
                        n247 = local write "STATUS"("Go to NEXT VECTOR" ("STATUS")) -> ()
                      }
                    }
                  }
                }
              }
            }
          }
        }
      }
      frame #2 {
      }
      frame #3 {
        n248 = Not Equal?(x=w610, y=w609) -> (x != y?=w608:bool)
        n249 = case shown="False" w608 {
          tunnel: w613 -> [_ w621]
          tunnel: w612 -> [_ w620]
          tunnel: [w614 w618] -> w611
          tunnel: w607 -> [w614 w615]
          frame #0 {
          }
          frame #1 {
            w616 = u16 1 items=["RAMP", "PAUSE", "MANUAL UP", "MANUAL DOWN", "ZERO"] ("Ramping Mode")
            n250 = call <userlib>:"Set Ramping Mode.vi"("error in"=w615, "Ramping Mode"=w616, "Communications Config"=w621) -> ("error out"=w619:T5)
            n251 = call <userlib>:"Set Ramping Mode.vi"("error in"=w619, "Ramping Mode"=w616, "Communications Config"=w620) -> ("error out"=w618:T5)
            n252 = local write "STATUS"("All Programmers are PAUSED. Set Ramping Mode to NEXT VECTOR to continue." ("STATUS")) -> ()
          }
        }
      }
      frame #4 {
        n253 = Not Equal?(x=w625, y=w627) -> (x != y?=w626:bool)
        n254 = case shown="False" w626 {
          tunnel: w630 -> [_ w639]
          tunnel: w629 -> [_ w638]
          tunnel: [w631 w634] -> w628
          tunnel: w624 -> [_ w637]
          tunnel: w623 -> [_ w636]
          tunnel: w622 -> [w631 w632]
          frame #0 {
          }
          frame #1 {
            w633 = u16 4 items=["RAMP", "PAUSE", "MANUAL UP", "MANUAL DOWN", "ZERO"] ("Ramping Mode")
            n255 = local write "STATUS"("Zeroing vector." ("STATUS")) -> ()
            n256 = call <userlib>:"Set Ramping Mode.vi"("error in"=w632, "Ramping Mode"=w633, "Communications Config"=w639) -> ("error out"=w642:T5)
            n257 = call <userlib>:"Set Ramping Mode.vi"("error in"=w642, "Ramping Mode"=w633, "Communications Config"=w638) -> ("error out"=w635:T5)
            n258 = call <userlib>:"Set Current Ramp Rate.vi"("Communications Config"=w639, "Ramp Rate (A/sec)"=w637, "error in"=w635) -> ("error out"=w640:T5)  [unwired: 2 in]
            n259 = call <userlib>:"Set Current Ramp Rate.vi"("Communications Config"=w638, "Ramp Rate (A/sec)"=w636, "error in"=w640) -> ("error out"=w634:T5)  [unwired: 2 in]
          }
        }
      }
    }
    n260 = local read "Continue Execution?"() -> (w253:bool)
  }
  n261 = case shown="0, Default" w30 {
    tunnel: w26 -> [w645 _ _]
    tunnel: w24 -> [w644 w648 w649]
    tunnel: [w643 w647 w649] -> w31
    tunnel: w25 -> [_ w646 _]
    frame #0 {
      n262 = call <userlib>:"430_TCP_Close.vi"("error in (no error)"=w644, "connection ID"=w645) -> ("error out"=w643:errorcluster)  [unwired: 1 out]
    }
    frame #1 {
      n263 = call <userlib>:"430_RS232_Close.vi"("error in (no error)"=w648, "VISA resource name"=w646) -> ("error out"=w647:errorcluster)  [unwired: 1 in]
    }
    frame #2 {
    }
  }
  n264 = case shown="0, Default" w29 {
    tunnel: w28 -> [w652 _ _]
    tunnel: w31 -> [w651 w655 w656]
    tunnel: [w650 w654 w656] -> w21
    tunnel: w27 -> [_ w653 _]
    frame #0 {
      n265 = call <userlib>:"430_TCP_Close.vi"("error in (no error)"=w651, "connection ID"=w652) -> ("error out"=w650:errorcluster)  [unwired: 1 out]
    }
    frame #1 {
      n266 = call <userlib>:"430_RS232_Close.vi"("error in (no error)"=w655, "VISA resource name"=w653) -> ("error out"=w654:errorcluster)  [unwired: 1 in]
    }
    frame #2 {
    }
  }
  "error out" <- w21
  n267 = local read "Magnetic Field Units"() -> (w48:u16)
  n268 = local read "Coordinate System"() -> (w49:u16)
  n269 = while {
    tunnel: "Starting index" -> [w664]
    tunnel: w23 -> [w670]
    tunnel: w22 -> [w671]
    tunnel: w48 -> [w672]
    tunnel: w49 -> [w673]
    tunnel: w46 -> [w676]
    tunnel: "Max Ramp Rate - Y Axis (A/s)" -> [w660]
    tunnel: "Max Ramp Rate - Z Axis (A/s)" -> [w659]
    tunnel: "Magnitude Limit (kG)" -> [w661]
    tunnel: "User defined Ramp Rate (T/min)" -> [w658]
    tunnel: "User defined Ramp Rate (T/min)" -> [w657]
    i -> [w663]
    stop <- w665 continue-if-true
    n270 = local read "Field Values"() -> (w667:string[][])
    n271 = Add(x=w664, y=w663) -> (x+y=w662:i32)
    n272 = while "Wait for NEXT VECTOR setting by operator." {
      tunnel: [w680] -> w675
      tunnel: w676 -> [w680]
      stop <- w681 continue-if-true
      w679 = u16 0 items=["NEXT VECTOR", "RAMPING", "HOLDING", "PAUSE", "ZERO"] ("Ramping Control")
      n273 = local read "Ramping Control"() -> (w682:u16)
      n274 = Not Equal?(x=w679, y=w682) -> (x != y?=w681:bool)
    }
    n275 = stacked-sequence {
      tunnel: w662 -> [w684 _ w690 _]
      frame #0 {
        (unwired) -2
        n276 = Subtract(x=w684, y=2) -> (x-y=w687:i32)
        n277 = Bundle(w687, -2) -> (w685:cluster{i32, i32})  [unwired: 1 in]
        n278 = property on="Field Values" class="Tbl (strict)"("Active Cell:Active Cell"=w685) -> ()  [unwired: 2 in, 2 out]
      }
      frame #1 {
        n279 = local read "Normal color"() -> (w688:u32)
        n280 = property on="Field Values" class="Tbl (strict)"("Active Cell:Cell Background Color"=w688) -> ()  [unwired: 2 in, 2 out]
      }
      frame #2 {
        n281 = Decrement(x=w690) -> (x-1=w689:i32)
        n282 = Bundle(w689, -2) -> (w692:cluster{i32, i32})  [unwired: 1 in]
        n283 = property on="Field Values" class="Tbl (strict)"("Active Cell:Active Cell"=w692) -> ()  [unwired: 2 in, 2 out]
      }
      frame #3 {
        n284 = property on="Field Values" class="Tbl (strict)"("Active Cell:Cell Background Color"="Highlight color") -> ()  [unwired: 2 in, 2 out]
      }
    }
    n285 = Index Array(array=w667, index (row)=w662) -> (element=w674:string[])  [unwired: 1 in]
    n286 = local write "Starting index"(w662) -> ()
    n287 = Add(x=1, y=w662) -> (x+y=w677:i32)
    n288 = Number To Decimal String(number=w677) -> (decimal integer string=w666:string)  [unwired: 1 in]
    n289 = stacked-sequence {
      tunnel: [_ w718] -> w668
      tunnel: [_ w717] -> w669
      tunnel: w675 -> [_ w713]
      tunnel: w674 -> [_ w712]
      tunnel: w673 -> [_ w711]
      tunnel: w672 -> [_ w710]
      tunnel: w671 -> [_ w709]
      tunnel: w670 -> [_ w708]
      tunnel: w666 -> [_ w707]
      tunnel: w661 -> [_ w705]
      tunnel: w660 -> [_ w704]
      tunnel: w659 -> [_ w699]
      tunnel: w658 -> [_ w703]
      tunnel: w657 -> [_ w702]
      frame #0 {
        w697 = u16 1 items=["NEXT VECTOR", "RAMPING", "HOLDING", "PAUSE", "ZERO"] ("Ramping Control")
        n290 = local write "Ramping Control"(w697) -> ()
      }
      frame #1 {
        n291 = call <userlib>:"Set 2D Next Vector_entwurf.vi"("Coordinate System"=w711, "Magnetic Field Units"=w710, 3:"User defined Ramp Rate (T/min)"=w702, "Magnitude Limit (kG)"=w705, "Y-Axis Communications Config"=w709, "Input Vector"=w712, "Z-Axis Communications Config"=w708, 10:"User defined Ramp Rate (T/min)"=w703, "Max Ramp Rate - Y Axis (A/s)"=w704, "error in"=w713, "Max Ramp Rate - Z Axis (A/s)"=w699) -> ("Y-Axis Ramp Rate (T/min)"=→"Current Ramp Rate Y (T/min)":dbl, "Within Limits?"=w718:bool, "Ramp Rate along Vector (T/min)"=→"Ramp Rate along Vector (T/min)":dbl, "Z-Axis Ramp Rate (T/min)"=→"Current Ramp Rate Z (T/min)":dbl, "All Instruments Responded?"=w717:bool, "error out"=w706:T5)  [unwired: 3 in]
        n292 = Concatenate Strings("Ramping to field vector " ("STATUS"), w707, "..." ("STATUS")) -> (w714:string)
        n293 = local write "error in"(w706) -> ()
        n294 = local write "STATUS"(w714) -> ()
      }
    }
    n295 = case shown="True" w668 {
      tunnel: w669 -> [_ w695]
      frame #0 {
        n296 = local write "STATUS"("Vector magnitude limt or maximum coil current exceeded. Vector ignored. VI halted." ("STATUS")) -> ()
      }
      frame #1 {
        n297 = case shown="True" w695 {
          frame #0 {
            n298 = local write "STATUS"("Not all programmers responded. VI halted." ("STATUS")) -> ()
          }
          frame #1 {
          }
        }
      }
    }
    n299 = Compound Arithmetic op=AND(w669, w668) -> (w665:bool)
    n300 = local write "Continue Execution?"(w665) -> ()
  }
